vi "PSW_03.vi"(0 "type":enum16{"AR-721H", "AR-821EF"}(ring), 2 "select":enum16{"Setup", "Search", "Release"}(ring), 7 "key":u8[](array[numeric]), 11 "error in":errorcluster) -> (4 "values":i32, 6 "found":bool, 15 "error out":errorcluster)   [LabVIEW 2011]
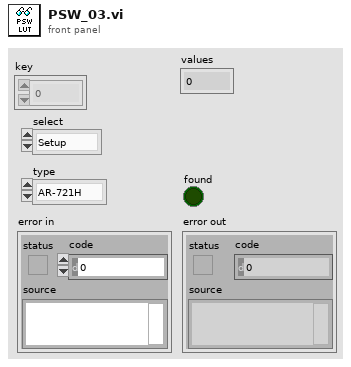
[diagram p1: front panel]
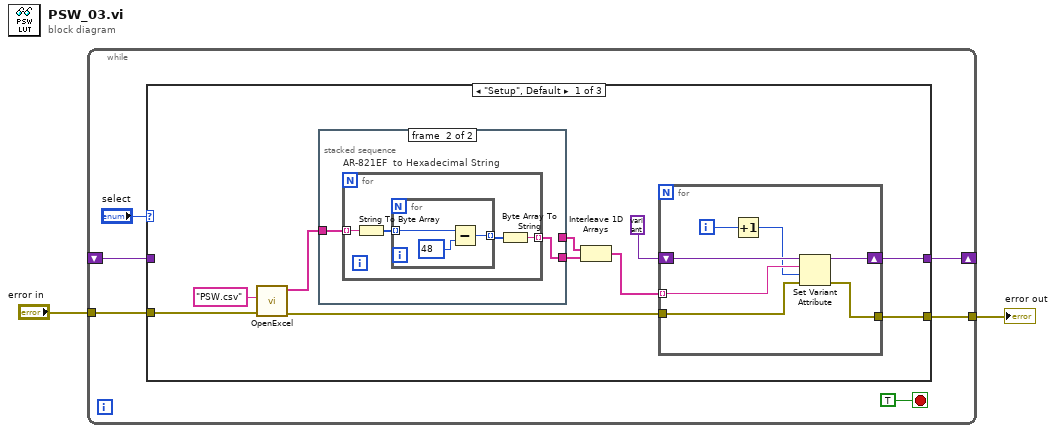
[diagram p0: block diagram]
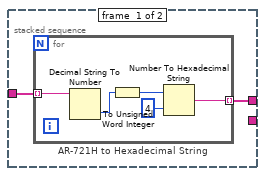
[diagram p2: hidden frame]
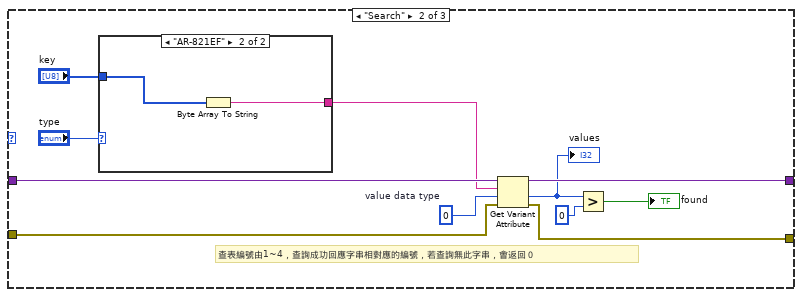
[diagram p3: hidden frame]
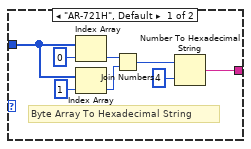
[diagram p4: hidden frame]
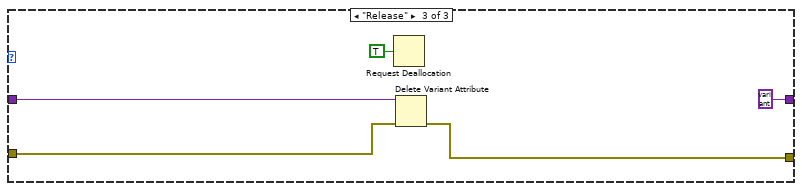
[diagram p5: hidden frame]
diagram:
  n1 = while {
    shift-right: [w8] -> _
    shift-left: _ -> [w7]
    tunnel: "error in" -> [w4]
    tunnel: [w3] -> w1
    stop <- TRUE stop-if-true
    n2 = case shown="\"Setup\", Default" "select" {
      tunnel: [w17 w50 variant ("variant")] -> w8
      tunnel: w7 -> [_ w51 w67]
      tunnel: w4 -> [w14 w45 w63]
      tunnel: [w12 w44 w64] -> w3
      frame "Setup", Default {
        n3 = call "OpenExcel.vi"("error in (no error)"=w14, "name or relative path"="PSW.csv") -> ("error out"=w13:errorcluster, "all rows"=w11:string[])  [unwired: 7 in, 1 out]
        n4 = stacked-sequence {
          tunnel: w11 -> [w20 w27]
          tunnel: [w19 _] -> w10
          tunnel: [_ w26] -> w9
          frame #0 {
            n5 = for "AR-721H to Hexadecimal String" {
              tunnel: w20 -> [w22] mode=indexing
              tunnel: [w21] -> w19 mode=indexing
              n6 = Decimal String To Number(string=w22) -> (number=w23:i32)  [unwired: 2 in, 1 out]
              n7 = To Unsigned Word Integer(number=w23) -> (unsigned 16bit integer=w24:u16)
              n8 = Number To Hexadecimal String(1:i16 4 ("width (-)"), 2:w24) -> (0:w21:string)
            }
          }
          frame #1 {
            n9 = for "AR-821EF  to Hexadecimal String" {
              tunnel: w27 -> [w29] mode=indexing
              tunnel: [w30] -> w26 mode=indexing
              n10 = String To Byte Array(string=w29) -> (unsigned byte array=w31:u8[])
              n11 = for {
                tunnel: w31 -> [w34] mode=indexing
                tunnel: [w32] -> w28 mode=indexing
                n12 = Subtract(x=w34, y=u8 48) -> (x-y=w32:u8)
              }
              n13 = Byte Array To String(unsigned byte array=w28) -> (string=w30:string)
            }
          }
        }
        n14 = Interleave 1D Arrays(w10, w9) -> (w16:string[])
        n15 = for {
          shift-right: [w40] -> w17
          shift-left: variant ("variant") -> [w41]
          tunnel: w16 -> [w39] mode=indexing
          tunnel: w13 -> [w36]
          tunnel: [w35] -> w12
          i -> [w37]
          n16 = Increment(x=w37) -> (x+1=w38:i32)
          n17 = Set Variant Attribute(Variant=w41, name=w39, value=w38, error in=w36) -> (Variant out=w40:variant, error out=w35:errorcluster)  [unwired: 1 out]
        }
      }
      frame "Search" {
        w52 = 0  # value data type
        # "查表編號由1~4，查詢成功回應字串相對應的編號，若查詢無此字串，會返回０"
        n18 = case shown="\"AR-821EF\"" "type" {
          tunnel: "key" -> [w60 w62]
          tunnel: [w59 w61] -> w48
          frame "AR-721H", Default {
            # "Byte Array To Hexadecimal String"
            n19 = Index Array(array=w60, index=0) -> (element=w54:u8)
            n20 = Index Array(array=w60, index=1) -> (element=w53:u8)
            n21 = Join Numbers(hi=w54, lo=w53) -> ((hi.lo)=w58:u16)
            n22 = Number To Hexadecimal String(1:i16 4 ("width (-)"), 2:w58) -> (0:w59:string)
          }
          frame "AR-821EF" {
            n23 = Byte Array To String(unsigned byte array=w62) -> (string=w61:string)
          }
        }
        n24 = Get Variant Attribute(Variant=w51, name=w48, default value (empty Variant)=w52, error in=w45) -> (duplicate Variant=w50:variant, value=w42:i32, error out=w44:errorcluster)  [unwired: 1 out]
        "values" <- w42
        n25 = Greater?(x=w42, y=0) -> (0:→"found":bool)
      }
      frame "Release" {
        n26 = Request Deallocation(TRUE ("flag")) -> ()
        n27 = Delete Variant Attribute(4:w63, 7:w67) -> (0:w64:errorcluster)  [unwired: 1 in, 2 out]
      }
    }
  }
  "error out" <- w1
